vi "Main.vi"() -> ()   [LabVIEW 2014]
doc: "This example shows a simulated RC (low-pass filter) circuit that illustrates the display non-ASCII text, particularly symbols common to science and engineering.\n\n<b>Showcase</b>\n- Displaying UFT-8 text\n- Displaying rich text\n- 2D plotting\n- Layout management\n\n\nCopyright (c) 2019 Sze Howe Koh.\nThis code is licensed under the MIT license."
uses:
  <vilib>/addons/LQ/Qwt/QwtPlot/Axis.ctl
  <vilib>/addons/LQ/Qt Widgets/QBoxLayout/Direction.ctl
  <vilib>/addons/LQ/LQ Core/QSize.ctl
  System Spec Widget/System Parameters.ctl
  Derived Params Widget/Derived Parameters.ctl
  <vilib>/addons/LQ/Qt Widgets/QWidget/resize.vi
  <vilib>/addons/LQ/Qt Widgets/QWidget/setVisible.vi
  <vilib>/addons/LQ/Qt Widgets/QWidget/setFont.vi
  <vilib>/addons/LQ/LQ Extras/LQChart/LQChart.lvclass
  <vilib>/addons/LQ/LQ Core/LQCoreEngine/LQCoreEngine.lvclass
  System Spec Widget/System Spec Widget.lvclass
  <vilib>/addons/LQ/Qwt/QwtPlot/QwtPlot.lvclass
  Derived Params Widget/Derived Params Widget.lvclass
  <vilib>/addons/LQ/Qt Widgets/QWidget/QWidget.lvclass
  <vilib>/addons/LQ/Qt Widgets/QBoxLayout/QBoxLayout.lvclass
  <vilib>/addons/LQ/Qt Widgets/QLabel/QLabel.lvclass
  <vilib>/addons/LQ/Qt GUI/QPixmap/QPixmap.lvclass
  <vilib>/addons/LQ/Qt GUI/QFont/QFont.lvclass
panel:
  in  "Stop Button":bool
  # "Prerequisite knowledge/experience\n- Basic LabVIEW programming\n- Example 4. Inheriting from a Widget from the \"Hello World - Introduction to Widgets\" series\n\nDescription\nThis example shows a simulated RC (low-pass filter) circuit that illustrates the display non-ASCII\ntext, particularly symbols common to science and engineering.\n\nShowcase\n- Displaying UFT-8 text\n- Displaying rich text\n- 2D plotting\n- Layout management"
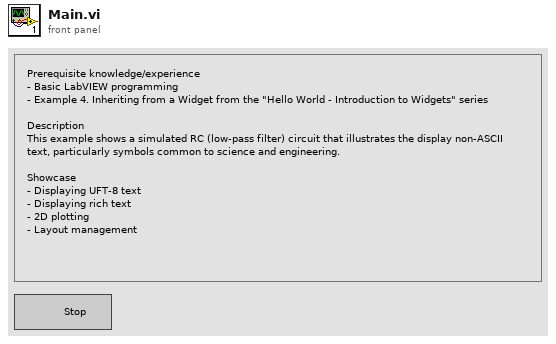
[diagram p1: front panel]
types:
  T1 = typedef "QSize.ctl" = cluster{"width":i32, "height":i32}
  T2 = typedef "QwtPlot.lvclass/Axis.ctl" = i32
  T3 = typedef "QBoxLayout.lvclass/Direction.ctl" = i32
  T4 = typedef "System Spec Widget.lvclass/System Parameters.ctl" = cluster{"Input Frequency [Hz]":i32, "Resistance [kOhm]":i32, "Capacitance [µF]":i32}
  T5 = typedef "Derived Params Widget.lvclass/Derived Parameters.ctl" = cluster{"Time Constant [ms]":dbl, "Angular Frequency [rad/s]":dbl, "Amplitude Response":dbl, "Phase Response [rad]":dbl}
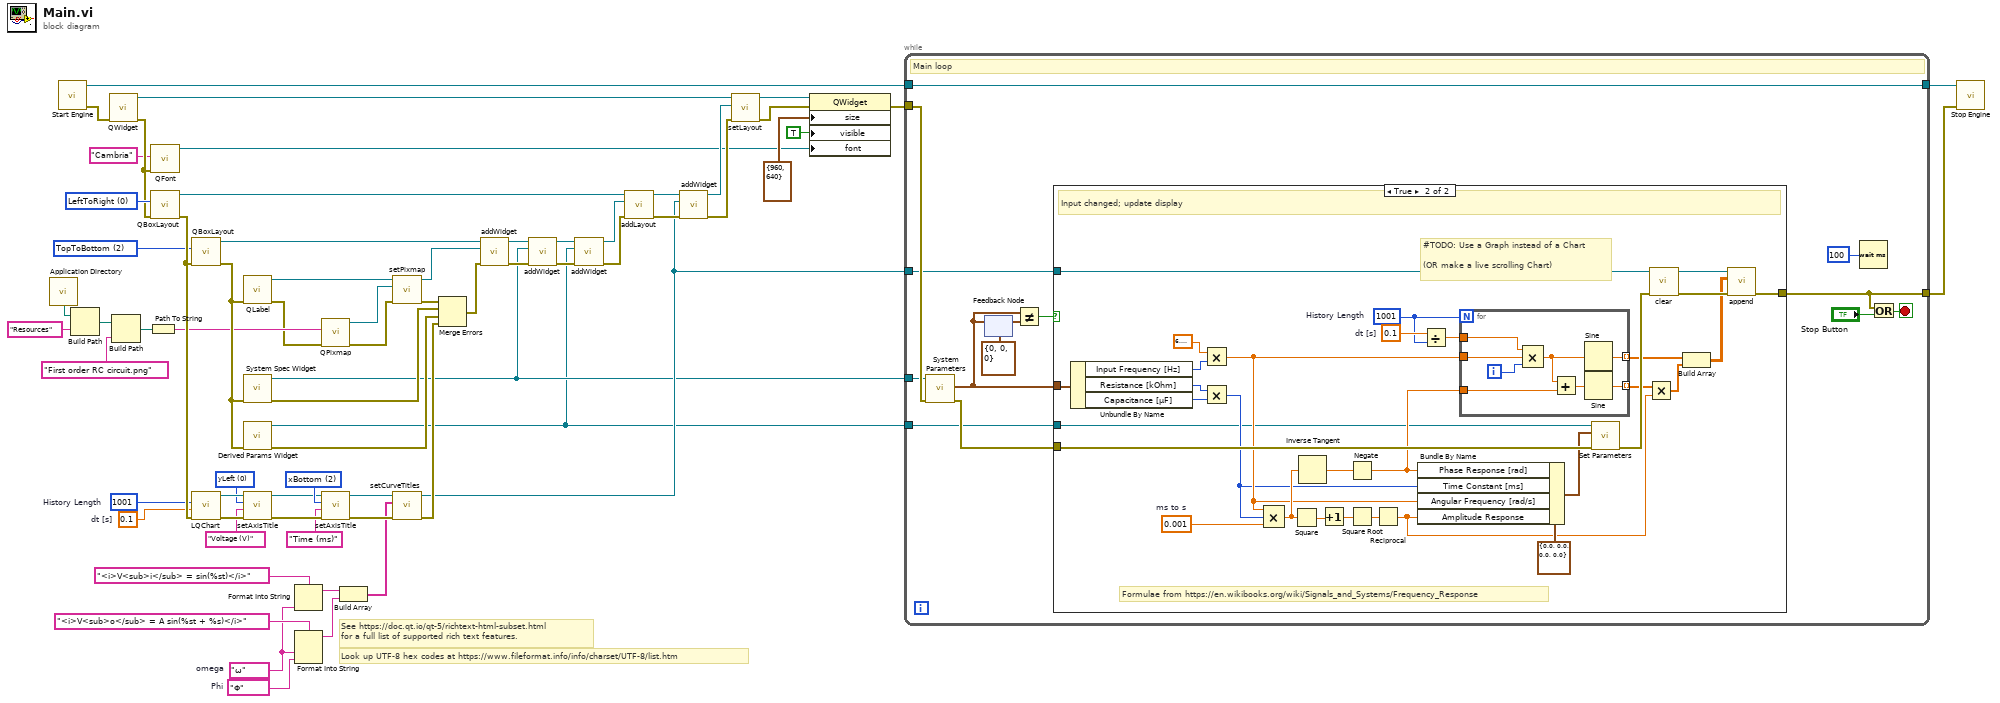
[diagram p0: block diagram]
diagram:
  w7 = "Φ"  # Phi
  w8 = "ω"  # omega
  w35 = T2 2 items=["yLeft", "yRight", "xBottom", "xTop"] ("axisId")
  w42 = T3 2 items=["LeftToRight", "RightToLeft", "TopToBottom", "BottomToTop"] ("direction")
  w43 = T3 0 items=["LeftToRight", "RightToLeft", "TopToBottom", "BottomToTop"] ("direction")
  w52 = T2 0 items=["yLeft", "yRight", "xBottom", "xTop"] ("axisId")
  w57 = 0.1  # dt [s]
  w58 = 1001  # History Length
  # "See https://doc.qt.io/qt-5/richtext-html-subset.html\nfor a full list of supported rich text features."
  # "Look up UTF-8 hex codes at https://www.fileformat.info/info/charset/UTF-8/list.htm"
  n1 = call <vilib>:"Application Directory.vi"() -> ("Application Directory"=w24:path)
  n2 = call <vilib>:"Start Engine.vi"() -> ("Error Out"=w44:errorcluster, "New Engine"=w50:refnum<class "LQCoreEngine.lvclass">)  [unwired: 10 in]
  n3 = Build Path(base path=w24, name or relative path="Resources") -> (appended path=w22:path)
  n4 = call <vilib>:"QWidget.vi"("Error In"=w44) -> ("Error Out"=w3:errorcluster, "New QWidget"=w49:refnum<class "QWidget.lvclass">)  [unwired: 9 in]
  n5 = Build Path(base path=w22, name or relative path="First order RC circuit.png" ("fileName")) -> (appended path=w20:path)
  n6 = Path To String(path=w20) -> (string=w19:string)
  n7 = call <vilib>:"QFont.vi"("Error In"=w3, "family"="Cambria") -> ("New QFont"=w1:refnum<class "QFont.lvclass">)  [unwired: 8 in, 1 out]
  n8 = call <vilib>:"QBoxLayout.vi"("Error In"=w3, "direction"=w43) -> ("Error Out"=w67:errorcluster, "New QBoxLayout"=w41:refnum<class "QBoxLayout.lvclass">)  [unwired: 8 in]
  n9 = call <vilib>:"QBoxLayout.vi"("Error In"=w67, "direction"=w42) -> ("Error Out"=w28:errorcluster, "New QBoxLayout"=w27:refnum<class "QBoxLayout.lvclass">)  [unwired: 8 in]
  n10 = call <vilib>:"LQChart.vi"("Error In"=w67, "xMultiplier"=w57, "historyLength"=w58) -> ("Error Out"=w54:errorcluster, "New LQChart"=w53:refnum<class "LQChart.lvclass">)  [unwired: 7 in]
  n11 = call <vilib>:"QLabel.vi"("Error In"=w28) -> ("Error Out"=w18:errorcluster, "New QLabel"=w25:refnum<class "QLabel.lvclass">)  [unwired: 9 in]
  n12 = call "System Spec Widget.vi"("Error In"=w28) -> ("Error Out"=w62:errorcluster, "New System Spec Widget"=w38:refnum<class "System Spec Widget.lvclass">)  [unwired: 9 in]
  n13 = call "Derived Params Widget.vi"("Error In"=w28) -> ("Error Out"=w63:errorcluster, "New Derived Params Widget"=w37:refnum<class "Derived Params Widget.lvclass">)  [unwired: 9 in]
  n14 = call <vilib>:"setAxisTitle.vi"("Error In"=w54, "title"="Voltage (V)", "axisId"=w52, "LQChart In"=w53) -> ("Error Out"=w59:errorcluster, "LQChart Out"=w34:refnum<class "LQChart.lvclass">)  [unwired: 6 in]
  n15 = Format Into String(format string="<i>V<sub>i</sub> = sin(%st)</i>", w8) -> (resulting string=w6:string)  [unwired: 2 in, 1 out]
  n16 = Format Into String(format string="<i>V<sub>o</sub> = A sin(%st + %s)</i>", w8, w7) -> (resulting string=w5:string)  [unwired: 2 in, 1 out]
  n17 = call <vilib>:"QPixmap.vi"("Error In"=w18, "fileName"=w19) -> ("Error Out"=w17:errorcluster, "New QPixmap"=w15:refnum<class "QPixmap.lvclass">)  [unwired: 8 in]
  n18 = call <vilib>:"setAxisTitle.vi"("Error In"=w59, "title"="Time (ms)", "axisId"=w35, "LQChart In"=w34) -> ("Error Out"=w60:errorcluster, "LQChart Out"=w33:refnum<class "LQChart.lvclass">)  [unwired: 6 in]
  n19 = Build Array(w6, w5) -> (w4:string[])
  n20 = call <vilib>:"setPixmap.vi"("Error In"=w17, "pixmap"=w15, "QLabel In"=w25) -> ("Error Out"=w12:errorcluster, "QLabel Out"=w16:refnum<class "QLabel.lvclass">)  [unwired: 7 in]
  n21 = call <vilib>:"setCurveTitles.vi"("Error In"=w60, "titles"=w4, "LQChart In"=w33) -> ("Error Out"=w61:errorcluster, "LQChart Out"=w46:refnum<class "LQChart.lvclass">)  [unwired: 7 in]
  n22 = Merge Errors(w12, w62, w63, w61) -> (w11:errorcluster)
  n23 = call <vilib>:"addWidget.vi"("Error In"=w11, "widget"=w16, "QBoxLayout In"=w27) -> ("Error Out"=w64:errorcluster, "QBoxLayout Out"=w26:refnum<class "QBoxLayout.lvclass">)  [unwired: 7 in]
  n24 = call <vilib>:"addWidget.vi"("Error In"=w64, "widget"=w38, "QBoxLayout In"=w26) -> ("Error Out"=w65:errorcluster, "QBoxLayout Out"=w47:refnum<class "QBoxLayout.lvclass">)  [unwired: 7 in]
  n25 = call <vilib>:"addWidget.vi"("Error In"=w65, "widget"=w37, "QBoxLayout In"=w47) -> ("Error Out"=w32:errorcluster, "QBoxLayout Out"=w39:refnum<class "QBoxLayout.lvclass">)  [unwired: 7 in]
  n26 = call <vilib>:"addLayout.vi"("Error In"=w32, "layout"=w39, "QBoxLayout In"=w41) -> ("Error Out"=w66:errorcluster, "QBoxLayout Out"=w40:refnum<class "QBoxLayout.lvclass">)  [unwired: 7 in]
  n27 = call <vilib>:"addWidget.vi"("Error In"=w66, "widget"=w46, "QBoxLayout In"=w40) -> ("Error Out"=w31:errorcluster, "QBoxLayout Out"=w45:refnum<class "QBoxLayout.lvclass">)  [unwired: 7 in]
  n28 = call <vilib>:"setLayout.vi"("Error In"=w31, "layout"=w45, "QWidget In"=w49) -> ("Error Out"=w30:errorcluster, "QWidget Out"=w48:refnum<class "QWidget.lvclass">)  [unwired: 7 in]
  n29 = property class="QWidget"(reference=w48, error in=w30, "size"=T1 {"width"=960, "height"=640}, "visible"=TRUE, "font"=w1) -> (error out=w29:errorcluster)  [unwired: 1 out]
  n30 = while {
    tunnel: w46 -> [w79]
    tunnel: w29 -> [w80]
    tunnel: w50 -> [w78]
    tunnel: [w78] -> w56
    tunnel: [w77] -> w55
    tunnel: w38 -> [w74]
    tunnel: w37 -> [w70]
    stop <- w75 stop-if-true
    # "Main loop"
    n31 = call "System Parameters.vi"("Error In"=w80, "System Spec Widget in"=w74) -> ("Error Out"=w81:errorcluster, "System Parameters"=w71:T4)  [unwired: 7 in, 1 out]
    n32 = feedback #1(T4 {"Input Frequency [Hz]"=0, "Resistance [kOhm]"=0, "Capacitance [µF]"=0} ("System Parameters")) -> (w73:T4)
    n33 = feedback-in #1(w71) -> ()
    n34 = Not Equal?(x=w71, y=w73) -> (x != y?=w72:bool)
    n35 = case shown="True" w72 {
      tunnel: w79 -> [_ w109]
      tunnel: [w82 w111] -> w77
      tunnel: w71 -> [_ w110]
      tunnel: w70 -> [_ w83]
      tunnel: w81 -> [w82 w113]
      frame False {
        # "Nothing new"
      }
      frame True {
        w86 = 0.1  # dt [s]
        w89 = 0.001  # ms to s
        w85 = 1001  # History Length
        # "Formulae from https://en.wikibooks.org/wiki/Signals_and_Systems/Frequency_Response"
        # "#TODO: Use a Graph instead of a Chart\n\n(OR make a live scrolling Chart)"
        # "Input changed; update display"
        n36 = Unbundle By Name(w110) -> ("Input Frequency [Hz]"=w103:i32, "Resistance [kOhm]"=w102:i32, "Capacitance [µF]"=w101:i32)
        n37 = Multiply(x=6.283185307179586, y=w103) -> (x*y=w94:dbl)
        n38 = Multiply(x=w102, y=w101) -> (x*y=w90:i32)
        n39 = Compound Arithmetic op=MULTIPLY(w94, w90, w89) -> (w97:dbl)
        n40 = Square(x=w97) -> (x^2=w100:dbl)
        n41 = Inverse Tangent(1:w97) -> (0:w96:dbl)
        n42 = Increment(x=w100) -> (x+1=w92:dbl)
        n43 = Negate(x=w96) -> (-x=w88:dbl)
        n44 = Square Root(x=w92) -> (sqrt(x)=w91:dbl)
        n45 = Reciprocal(x=w91) -> (1/x=w93:dbl)
        n46 = Bundle By Name(cluster=T5 {"Time Constant [ms]"=0.0, "Angular Frequency [rad/s]"=0.0, "Amplitude Response"=0.0, "Phase Response [rad]"=0.0} ("Derived Parameters"), "Phase Response [rad]"=w88, "Time Constant [ms]"=w90, "Angular Frequency [rad/s]"=w94, "Amplitude Response"=w93) -> (w87:T5)
        n47 = Divide(x=w86, y=w85) -> (x/y=w84:dbl)
        n48 = for {
          N: w85 -> [_]
          tunnel: [w118] -> w105 mode=indexing
          tunnel: [w117] -> w98 mode=indexing
          tunnel: w94 -> [w116]
          tunnel: w88 -> [w115]
          tunnel: w84 -> [w114]
          i -> [w121]
          n49 = Compound Arithmetic op=MULTIPLY(w114, w116, w121) -> (w120:dbl)
          n50 = Add(x=w120, y=w115) -> (x+y=w119:dbl)
          n51 = Sine(x=w120) -> (sin(x)=w118:dbl)
          n52 = Sine(x=w119) -> (sin(x)=w117:dbl)
        }
        n53 = call "Set Parameters.vi"("Error In"=w113, "Derived Parameters"=w87, "Derived Params Widget in"=w83) -> ("Error Out"=w112:errorcluster)  [unwired: 7 in, 1 out]
        n54 = Multiply(x=w98, y=w93) -> (x*y=w99:dbl[])
        n55 = call <vilib>:"clear.vi"("Error In"=w112, "LQChart In"=w109) -> ("Error Out"=w107:errorcluster, "LQChart Out"=w108:refnum<class "LQChart.lvclass">)  [unwired: 8 in]
        n56 = Build Array(w105, w99) -> (w106:dbl[][])
        n57 = call <vilib>:"append.vi"("Error In"=w107, "values"=w106, "LQChart In"=w108) -> ("Error Out"=w111:errorcluster)  [unwired: 7 in, 1 out]
      }
    }
    n58 = Wait (ms)(milliseconds to wait=u32 100 ("millisecond multiple")) -> ()  [unwired: 1 out]
    n59 = Or(x=w77, y="Stop Button") -> (x .or. y?=w75:bool)
  }
  n60 = call <vilib>:"Stop Engine.vi"("Error In"=w55, "LQCoreEngine"=w56) -> ()  [unwired: 9 in, 1 out]
